vi "Remote_______3.vi"() -> ()   [LabVIEW 2020]
uses:
  <vilib>/ReMiSYS Technology/L4VMX TitanQuad/TitanQuad.lvclass
  <vilib>/ReMiSYS Technology/L4VMX TitanQuad/Motor ID.ctl
  <vilib>/ReMiSYS Technology/L4VMX VMXpi/Type Def/VMX Channel Index.ctl
  <vilib>/ReMiSYS Technology/L4VMX VMXpi/L4VMX.lvlib
  <vilib>/ReMiSYS Technology/RemoteToolkit/Receiver/Receiver.lvclass
  <vilib>/ReMiSYS Technology/L4VMX VMXpi/Digital Input/Digital Input.lvclass
  stu.ctl
  <vilib>/ReMiSYS Technology/L4VMX VMXpi/PWM Generator/PWM Generator.lvclass
  <vilib>/ReMiSYS Technology/L4VMX VMXpi/Utilities/Utilities.lvclass
  <vilib>/ReMiSYS Technology/L4VMX VMXpi/Digital Output/Digital Output.lvclass
panel:
  in  "stop 2":bool
  out "------":dbl[](array[numeric])
  out "motor speed":dbl[](array[numeric])
  out "data":T1
  out "Counter Value":i32
  in  "stop":bool
  out "Stop0":bool
  out "Error Out":errorcluster
  in  "Stop":bool
  out "Received?":bool
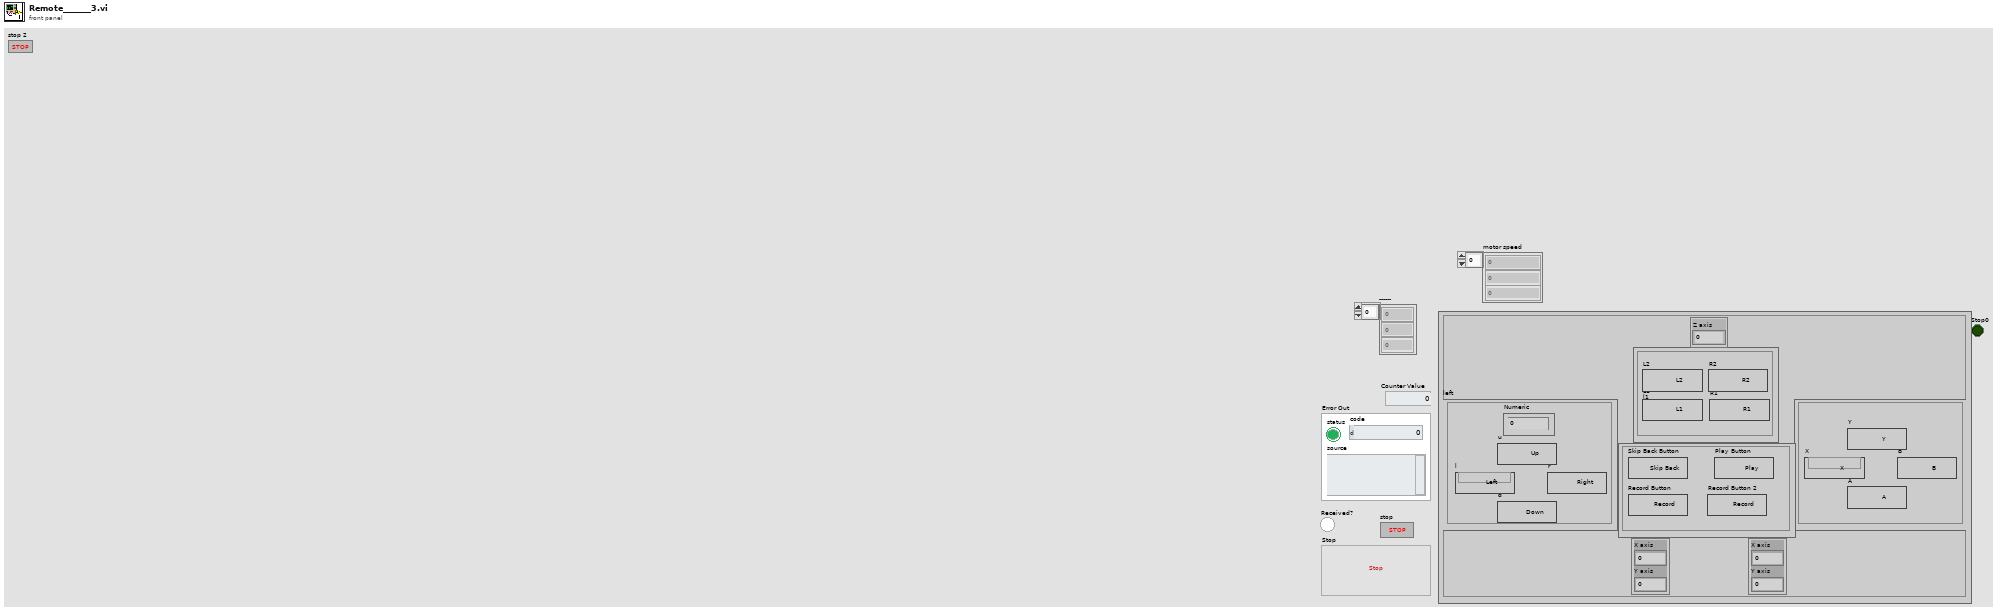
[diagram p1: front panel]
types:
  T1 = typedef "stu.ctl" = cluster{"Top Button":cluster{"L1\nl1":bool, "L2":bool, "R1":bool, "R2":bool}, "Left axis ":cluster{"X axis":i32, "Y axis":i32}, "Right axis  ":cluster{"X axis":i32, "Y axis":i32}, "right":cluster{"A":bool, "B":bool, "X":bool, "Y":bool}, "middle":cluster{"Skip Back Button":bool, "Play Button":bool, "Record Button":bool, "Record Button 2":bool}, "left":cluster{"d":bool, "r":bool, "l":bool, "u":bool, "Numeric":i32}, "top  z":cluster{"Z axis":i32}}
  T2 = typedef "L4VMX.lvlib/VMX Channel Index.ctl" = enum16{"0", "1", "2", "3", "4", "5", "6", "7", "8", "9", "10", "11", "12", "13", "14", "15", "16", "17", "18", "19", "20", "21", "22", "23", "24", "25", "26", "27", "28", "29", "30", "31", "32", "33"}
  T3 = typedef "TitanQuad.lvlib/TitanQuad.lvclass/Motor ID.ctl" = enum16{"M0", "M1", "M2", "M3"}
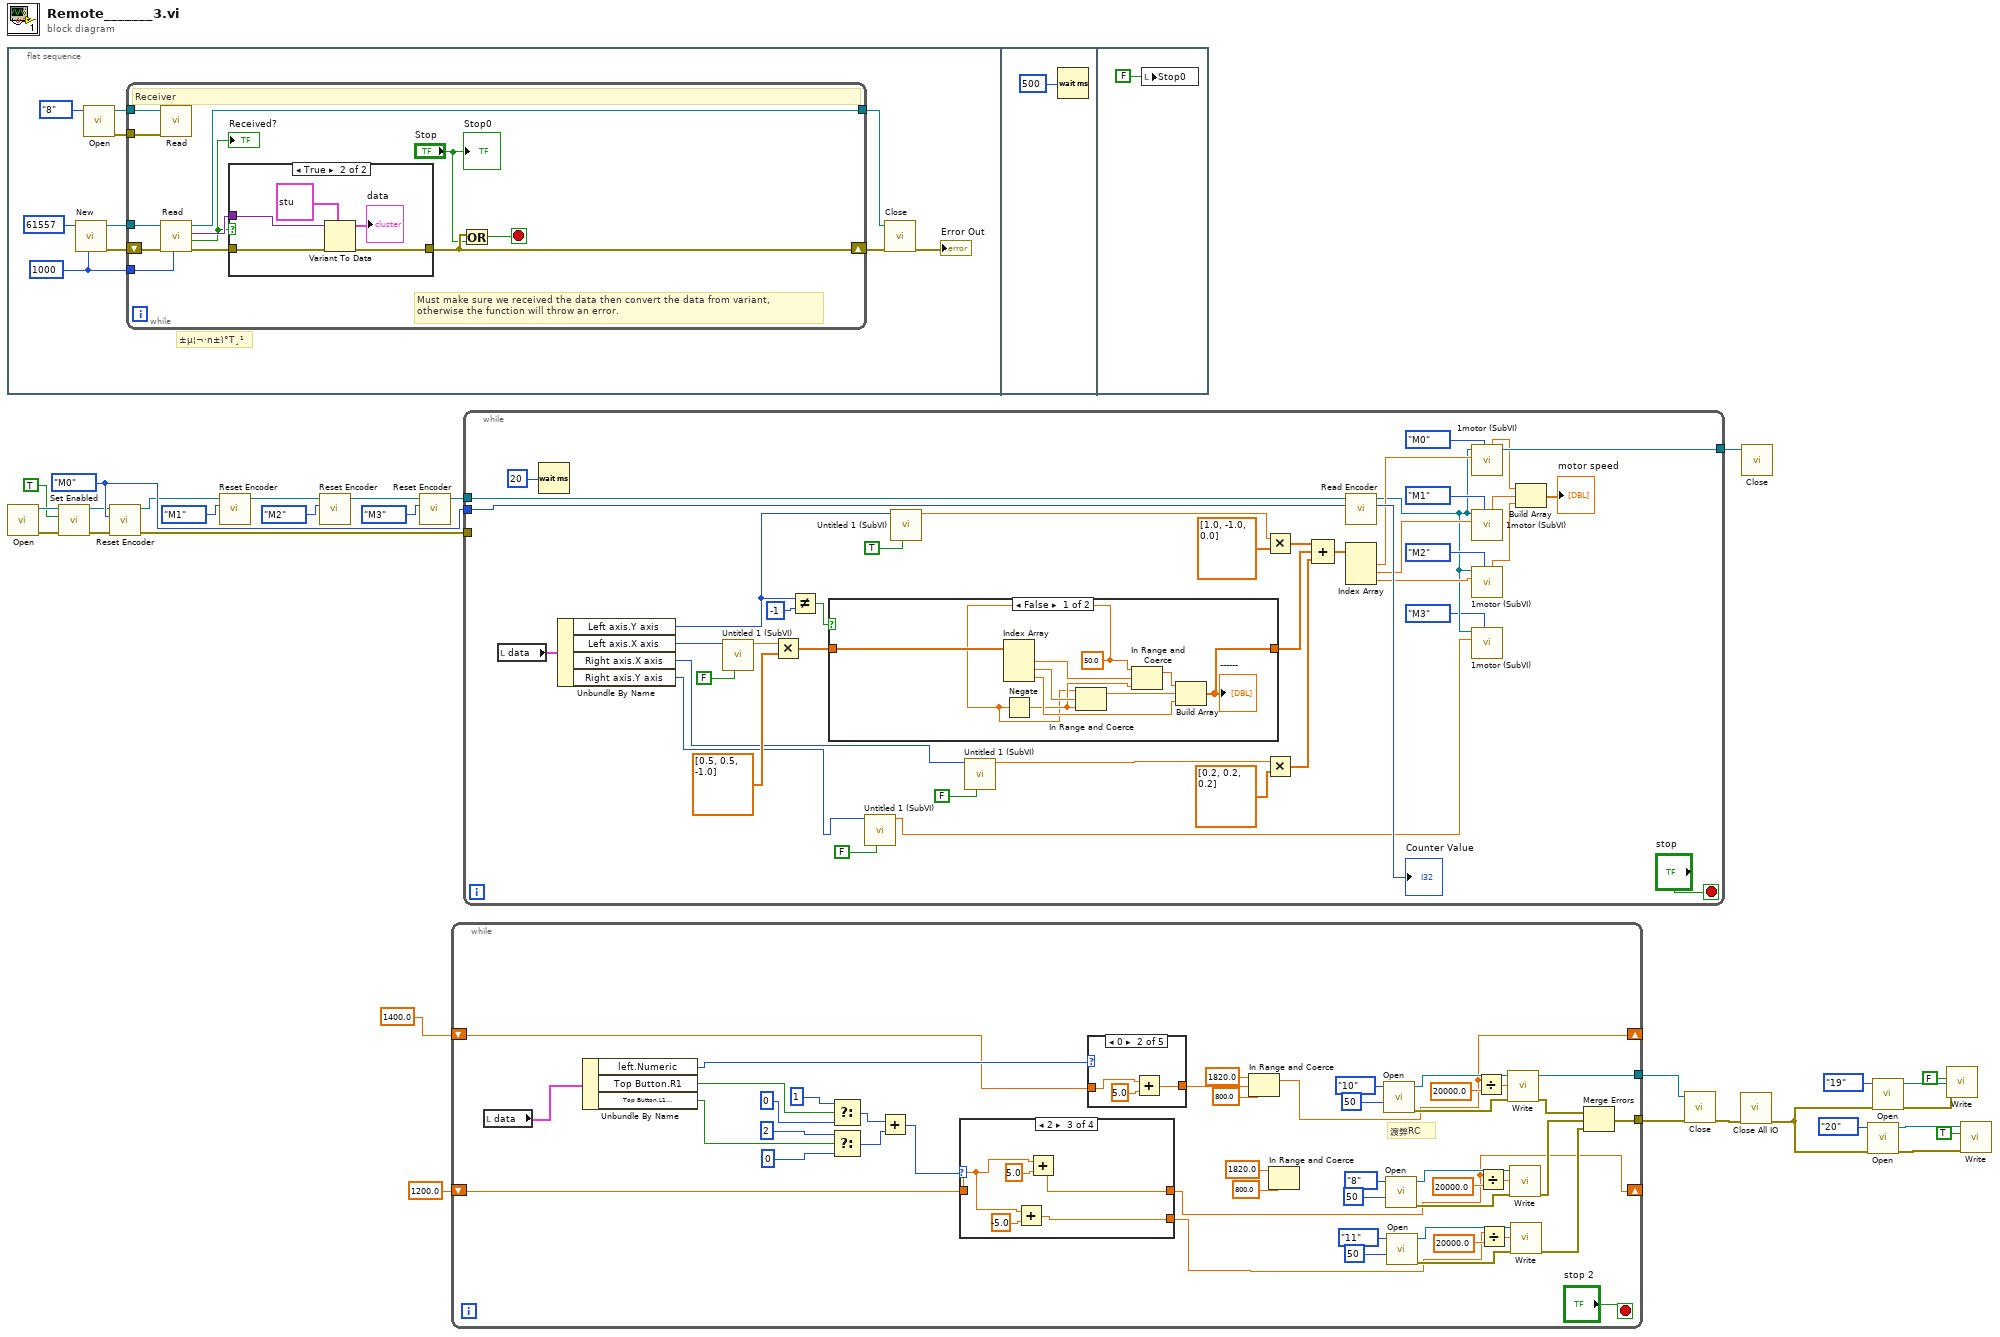
[diagram p0: block diagram]
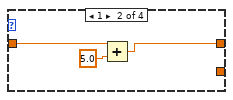
[diagram p3: hidden frame]
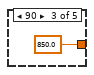
[diagram p6: hidden frame]
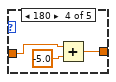
[diagram p7: hidden frame]
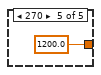
[diagram p8: hidden frame]
diagram:
  w26 = Motor_ID."M0" ("Motor ID")
  n1 = flat-sequence {
    frame #0 {
      w35 = 1000 ("Timeout ms (25000)")
      # "±µ¦¬·n±ì°T¸¹"
      n2 = call <vilib>:"New.vi"("Timeout ms (25000)"=w35, "Port (61557)"=u16 61557) -> ("Error Out"=w39:errorcluster, "Receiver Ref."=w38:refnum<class "Receiver.lvclass">)  [unwired: 8 in]
      n3 = call <vilib>:"Open.vi"("VMX Channel Index"=VMX_Channel_Index."8") -> ("Error Out"=w30:errorcluster, "Digital Input Object"=w31:refnum<class "Digital Input.lvclass">)  [unwired: 9 in]
      n4 = while {
        shift-right: [w44] -> w37
        shift-left: w39 -> [w51]
        tunnel: w38 -> [w50]
        tunnel: [w49] -> w36
        tunnel: w35 -> [w48]
        tunnel: w31 -> [w42]
        tunnel: w30 -> [w41]
        stop <- w47 stop-if-true
        # "Must make sure we received the data then convert the data from variant,\notherwise the function will throw an error."
        # "Receiver"
        n5 = call <vilib>:"Read.vi"("Error In"=w41, "Digital Input Object"=w42) -> ()  [unwired: 7 in, 3 out]
        n6 = call <vilib>:"Read.vi"("Timeout ms (1000)"=w48, "Error In"=w51, "Receiver Ref."=w50) -> ("Error Out"=w46:errorcluster, "Received?"=w43:bool, "Value"=w45:variant, "Receiver Ref."=w49:refnum<class "Receiver.lvclass">)  [unwired: 5 in]
        "Received?" <- w43
        n7 = case shown="True" w43 {
          tunnel: w46 -> [w52 w57]
          tunnel: w45 -> [_ w56]
          tunnel: [w52 w55] -> w44
          frame False {
          }
          frame True {
            n8 = Variant To Data(error in=w57, type=T1 {"Top Button"={"L1\nl1"=FALSE, "L2"=FALSE, "R1"=FALSE, "R2"=FALSE}, "Left axis "={"X axis"=0, "Y axis"=0}, "Right axis  "={"X axis"=0, "Y axis"=0}, "right"={"A"=FALSE, "B"=FALSE, "X"=FALSE, "Y"=FALSE}, "middle"={"Skip Back Button"=FALSE, "Play Button"=FALSE, "Record Button"=FALSE, "Record Button 2"=FALSE}, "left"={"d"=FALSE, "r"=FALSE, "l"=FALSE, "u"=FALSE, "Numeric"=0}, "top  z"={"Z axis"=0}} ("Cluster"), Variant=w56) -> (data=→"data":T1, error out=w55:errorcluster)
          }
        }
        n9 = Or(x=w44, y="Stop") -> (x .or. y?=w47:bool)
        "Stop0" <- "Stop"
      }
      n10 = call <vilib>:"Close.vi"("Error In"=w37, "Receiver Ref."=w36) -> ("Error Out"=→"Error Out":errorcluster)  [unwired: 9 in]
    }
    frame #1 {
      n11 = Wait (ms)(milliseconds to wait=u32 500) -> ()  [unwired: 1 out]
    }
    frame #2 {
      n12 = local write "Stop0"(FALSE ("Stop")) -> ()
    }
  }
  n13 = call <vilib>:"Open.vi"() -> ("Error Out"=w22:errorcluster, "TitanQuad Object"=w29:refnum<class "TitanQuad.lvclass">)  [unwired: 10 in]
  n14 = call <vilib>:"Set Enabled.vi"("Error In"=w22, "Enable"=TRUE, "TitanQuad Object"=w29) -> ("Error Out"=w21:errorcluster, "TitanQuad Object"=w25:refnum<class "TitanQuad.lvclass">)  [unwired: 7 in]
  n15 = call <vilib>:"Reset Encoder.vi"("Error In"=w21, "Motor ID"=w26, "TitanQuad Object"=w25) -> ("Error Out"=w20:errorcluster, "TitanQuad Object"=w24:refnum<class "TitanQuad.lvclass">)  [unwired: 7 in]
  n16 = call <vilib>:"Reset Encoder.vi"("Motor ID"=Motor_ID."M1", "TitanQuad Object"=w24) -> ("TitanQuad Object"=w19:refnum<class "TitanQuad.lvclass">)  [unwired: 8 in, 1 out]
  n17 = call <vilib>:"Reset Encoder.vi"("Motor ID"=Motor_ID."M2", "TitanQuad Object"=w19) -> ("TitanQuad Object"=w15:refnum<class "TitanQuad.lvclass">)  [unwired: 8 in, 1 out]
  n18 = call <vilib>:"Reset Encoder.vi"("Motor ID"=Motor_ID."M3", "TitanQuad Object"=w15) -> ("TitanQuad Object"=w16:refnum<class "TitanQuad.lvclass">)  [unwired: 8 in, 1 out]
  n19 = while {
    tunnel: [w95] -> w4
    shift-right: [w64] -> _
    shift-left: 1200.0 ("upper limit") -> [w72]
    shift-right: [w90] -> _
    shift-left: 1400.0 ("upper limit") -> [w91]
    tunnel: [w89] -> w1
    stop <- "stop 2" stop-if-true
    # "渡弊RC"
    n20 = local read "data"() -> (w94:T1)
    n21 = Unbundle By Name(w94) -> ("left.Numeric"=w92:i32, "Top Button.R1"=w88:bool, "Top Button.L1\nl1"=w87:bool)
    n22 = Select(t=1, s=w88, f=0) -> (s? t:f=w82:i32)
    n23 = Select(t=2, s=w87, f=0) -> (s? t:f=w81:i32)
    n24 = Add(x=w82, y=w81) -> (x+y=w80:i32)
    n25 = case shown="2" w80 {
      tunnel: [w106 w107 w113 w115] -> w64
      tunnel: w72 -> [w106 w108 w111 w115]
      tunnel: [_ _ w110 _] -> w63
      frame 0, Default {
      }
      frame 1 {
        n26 = Add(x=w108, y=5.0) -> (x+y=w107:dbl)
      }
      frame 2 {
        n27 = Add(x=w111, y=-5.0) -> (x+y=w110:dbl)
        n28 = Add(x=w111, y=5.0) -> (x+y=w113:dbl)
      }
      frame 3 {
      }
    }
    n29 = case shown="0" w92 {
      tunnel: [w116 w118 850.0 ("y") w122 1200.0 ("y")] -> w97
      tunnel: w91 -> [w116 w117 _ w121 _]
      frame -1, Default {
      }
      frame 0 {
        n30 = Add(x=w117, y=5.0) -> (x+y=w118:dbl)
      }
      frame 90 {
      }
      frame 180 {
        n31 = Add(x=w121, y=-5.0) -> (x+y=w122:dbl)
      }
      frame 270 {
      }
    }
    n32 = In Range and Coerce(upper limit=1820.0, x=w97, lower limit=800.0) -> (coerced(x)=w90:dbl)  [unwired: 1 out]
    n33 = In Range and Coerce(upper limit=1820.0, lower limit=800.0) -> (x=w61:dbl)  [unwired: 2 out]
    n34 = call <vilib>:"Open.vi"("Frequency(Hz)"=u32 50, "VMX Channel Index"=VMX_Channel_Index."10") -> ("Error Out"=w99:errorcluster, "PWM Generator Object"=w100:refnum<class "PWM Generator.lvclass">)  [unwired: 8 in]
    n35 = call <vilib>:"Open.vi"("Frequency(Hz)"=u32 50, "VMX Channel Index"=VMX_Channel_Index."8") -> ("Error Out"=w74:errorcluster, "PWM Generator Object"=w75:refnum<class "PWM Generator.lvclass">)  [unwired: 8 in]
    n36 = call <vilib>:"Open.vi"("Frequency(Hz)"=u32 50, "VMX Channel Index"=VMX_Channel_Index."11") -> ("Error Out"=w71:errorcluster, "PWM Generator Object"=w70:refnum<class "PWM Generator.lvclass">)  [unwired: 8 in]
    n37 = Divide(x=w90, y=20000.0) -> (x/y=w105:dbl)
    n38 = Divide(x=w64, y=20000.0) -> (x/y=w79:dbl)
    n39 = Divide(x=w63, y=20000.0) -> (x/y=w66:dbl)
    n40 = call <vilib>:"Write.vi"("Error In"=w99, "Duty Cycle(0~1)"=w105, "PWM Generator Object"=w100) -> ("Error Out"=w103:errorcluster, "PWM Generator Object"=w89:refnum<class "PWM Generator.lvclass">)  [unwired: 7 in]
    n41 = call <vilib>:"Write.vi"("Error In"=w74, "Duty Cycle(0~1)"=w79, "PWM Generator Object"=w75) -> ("Error Out"=w73:errorcluster)  [unwired: 7 in, 1 out]
    n42 = call <vilib>:"Write.vi"("Error In"=w71, "Duty Cycle(0~1)"=w66, "PWM Generator Object"=w70) -> ("Error Out"=w65:errorcluster)  [unwired: 7 in, 1 out]
    n43 = Merge Errors(w103, w73, w65) -> (w95:errorcluster)
  }
  n44 = while {
    tunnel: w16 -> [w148]
    tunnel: [w165] -> w27
    tunnel: w20 -> [_]
    tunnel: w26 -> [w157]
    stop <- "stop" stop-if-true
    n45 = local read "data"() -> (w161:T1)
    n46 = Wait (ms)(milliseconds to wait=u32 20) -> ()  [unwired: 1 out]
    n47 = Unbundle By Name(w161) -> ("Left axis.Y axis"=w133:i32, "Left axis.X axis"=w159:i32, "Right axis.X axis"=w136:i32, "Right axis.Y axis"=w126:i32)
    n48 = call "Untitled 1 (SubVI).vi"("Boolean"=FALSE, "Y axis"=w159) -> ("Numeric"=w152:dbl)  [unwired: 9 in]
    n49 = Multiply(x=w152, y=dbl[] [0.5, 0.5, -1.0]) -> (x*y=w129:dbl[])
    n50 = Not Equal?(x=w133, y=-1) -> (x != y?=w130:bool)
    n51 = case shown="False" w130 {
      tunnel: w129 -> [w168 w175]
      tunnel: [w167 w175] -> w128
      frame False {
        w166 = 50.0
        n52 = Index Array(array=w168) -> (element #1=w173:dbl, element #2=w171:dbl, element #3=w174:dbl)  [unwired: 3 in]
        n53 = Negate(x=w166) -> (-x=w169:dbl)
        n54 = In Range and Coerce(upper limit=w166, x=w171, lower limit=w169) -> (coerced(x)=w170:dbl)  [unwired: 1 out]
        n55 = In Range and Coerce(upper limit=w166, x=w173, lower limit=w169) -> (coerced(x)=w172:dbl)  [unwired: 1 out]
        n56 = Build Array(w172, w170, w174) -> (w167:dbl[])
        "------" <- w167
      }
      frame True {
      }
    }
    n57 = call "Untitled 1 (SubVI).vi"("Boolean"=FALSE, "Y axis"=w126) -> ("Numeric"=w125:dbl)  [unwired: 9 in]
    n58 = call "Untitled 1 (SubVI).vi"("Boolean"=TRUE, "Y axis"=w133) -> ("Numeric"=w154:dbl)  [unwired: 9 in]
    n59 = call "Untitled 1 (SubVI).vi"("Boolean"=FALSE, "Y axis"=w136) -> ("Numeric"=w139:dbl)  [unwired: 9 in]
    n60 = Multiply(x=w154, y=dbl[] [1.0, -1.0, 0.0]) -> (x*y=w150:dbl[])
    n61 = Multiply(x=w139, y=dbl[] [0.2, 0.2, 0.2]) -> (x*y=w135:dbl[])
    n62 = Compound Arithmetic op=ADD(w150, w128, w135) -> (w144:dbl[])
    n63 = call <vilib>:"Read Encoder.vi"("Motor ID"=w157, "TitanQuad Object"=w148) -> ("Counter Value"=→"Counter Value":i32, "TitanQuad Object"=w132:refnum<class "TitanQuad.lvclass">)  [unwired: 7 in, 1 out]
    n64 = Index Array(array=w144) -> (element #1=w147:dbl, element #2=w146:dbl, element #3=w145:dbl)  [unwired: 3 in]
    n65 = call "1motor (SubVI).vi"("Motor ID"=Motor_ID."M0", "Numeric"=w147, "TitanQuad in"=w132) -> ("TitanQuad out"=w165:refnum<class "TitanQuad.lvclass">, "coerced(x)"=w143:dbl)  [unwired: 6 in, 1 out]
    n66 = call "1motor (SubVI).vi"("Motor ID"=Motor_ID."M1", "Numeric"=w146, "TitanQuad in"=w132) -> ("coerced(x)"=w142:dbl)  [unwired: 6 in, 2 out]
    n67 = call "1motor (SubVI).vi"("Motor ID"=Motor_ID."M2", "Numeric"=w145, "TitanQuad in"=w132) -> ("coerced(x)"=w141:dbl)  [unwired: 6 in, 2 out]
    n68 = call "1motor (SubVI).vi"("Motor ID"=Motor_ID."M3", "Numeric"=w125, "TitanQuad in"=w132) -> ()  [unwired: 6 in, 3 out]
    n69 = Build Array(w143, w142, w141) -> (→"motor speed":dbl[])
  }
  n70 = call <vilib>:"Close.vi"("Error In"=w4, "PWM Generator Object"=w1) -> ("Error Out"=w9:errorcluster)  [unwired: 9 in]
  n71 = call <vilib>:"Close All IO.vi"("Error In"=w9) -> ("Error Out"=w10:errorcluster)  [unwired: 10 in]
  n72 = call <vilib>:"Close.vi"("TitanQuad Object"=w27) -> ()  [unwired: 10 in, 1 out]
  n73 = call <vilib>:"Open.vi"("Error In"=w10, "VMX Channel Index"=VMX_Channel_Index."20") -> ("Error Out"=w12:errorcluster, "Digital Output Object"=w11:refnum<class "Digital Output.lvclass">)  [unwired: 8 in]
  n74 = call <vilib>:"Open.vi"("Error In"=w10, "VMX Channel Index"=VMX_Channel_Index."19") -> ("Error Out"=w14:errorcluster, "Digital Output Object"=w13:refnum<class "Digital Output.lvclass">)  [unwired: 8 in]
  n75 = call <vilib>:"Write.vi"("Error In"=w14, "Value"=FALSE, "Digital Output Object"=w13) -> ()  [unwired: 7 in, 2 out]
  n76 = call <vilib>:"Write.vi"("Error In"=w12, "Value"=TRUE, "Digital Output Object"=w11) -> ()  [unwired: 7 in, 2 out]
